vi "Main.vi"() -> ()   [LabVIEW 2017]
uses:
  types/Data Share Type.ctl
  E:/UPWORK/labview-offline-maps/labview/dll/OfflineMaps.Core.dll
  dll/OfflineMaps.Core.dll
  E:/UPWORK/labview-offline-maps/labview/dll/OfflineMaps.Controls.dll
  dll/OfflineMaps.Controls.dll
panel:
  in  "Load Button":bool
  in  "Temperature Alarm":dbl=25.0 caption="Alarm when temperature over, C"
  in  "Track file":path caption="Track file path:"
  in  "Map folder":path caption="Map folder path:"
  in  "Exit Button":bool
  in  "OfflineMapControl":refnum<k24>(container)
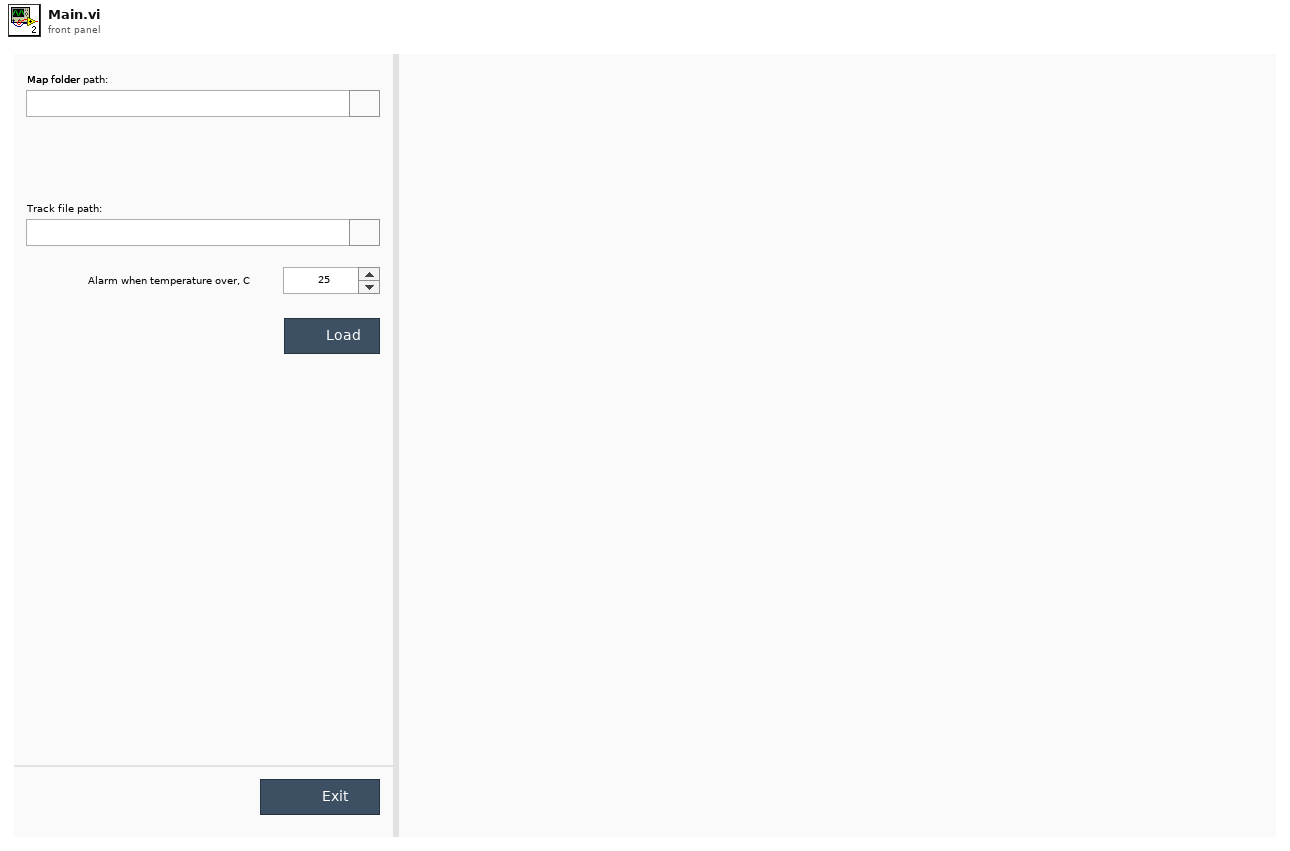
[diagram p1: front panel]
types:
  T1 = typedef "Data Share Type.ctl" = cluster{"Map folder":path, "Track file":path, "Latitude, deg:":dbl, "Longitude, deg:":dbl}
  T2 = cluster{"Warning":bool, "Caption":string, "Latitude_deg":dbl, "Longitude_deg":dbl, "Altitude_m":dbl, "Speed_m_s":dbl, "Temperature_C":dbl}[]
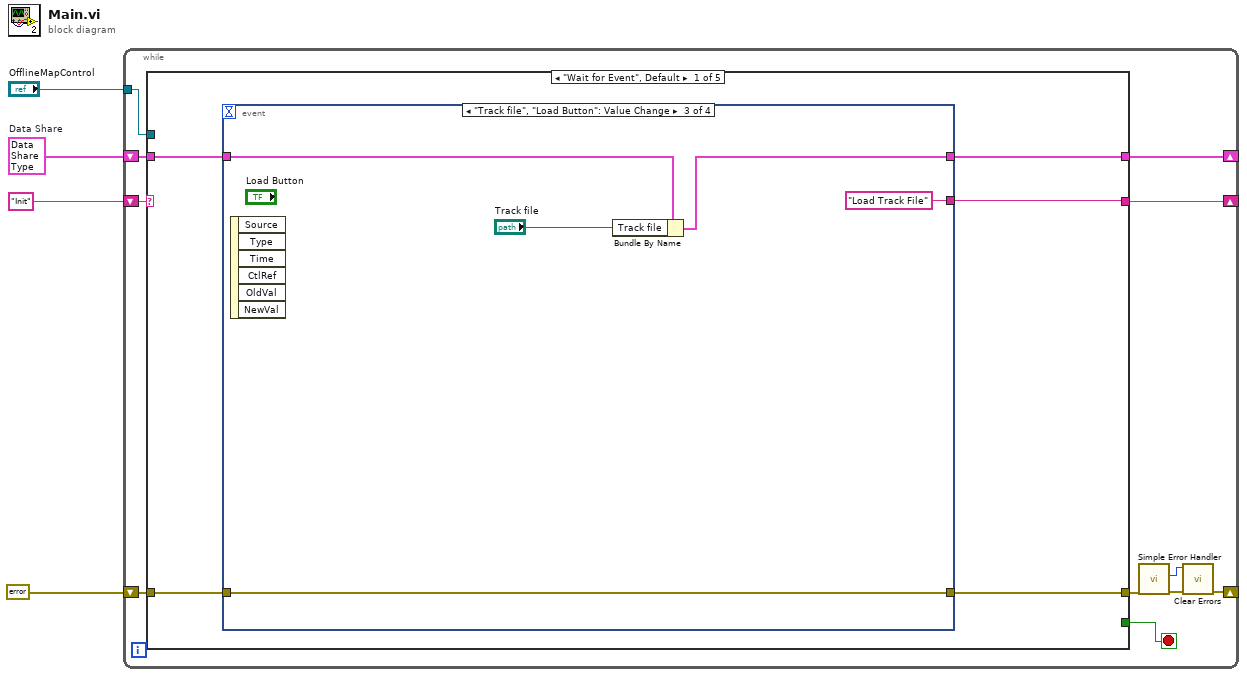
[diagram p0: block diagram]
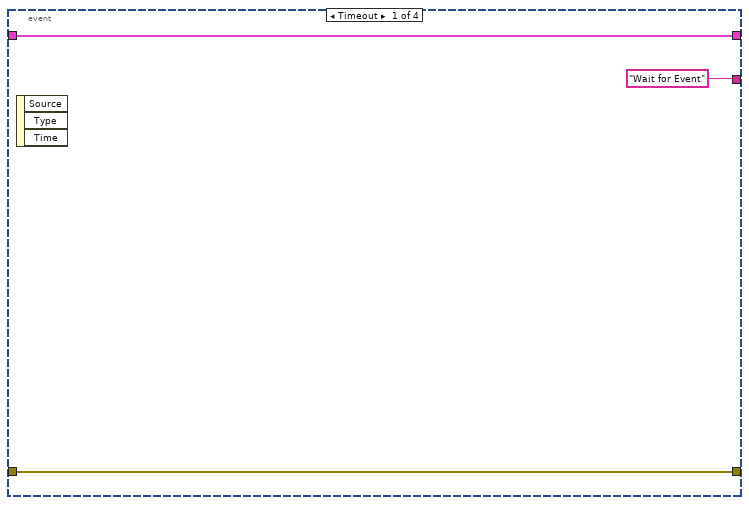
[diagram p2: hidden frame]
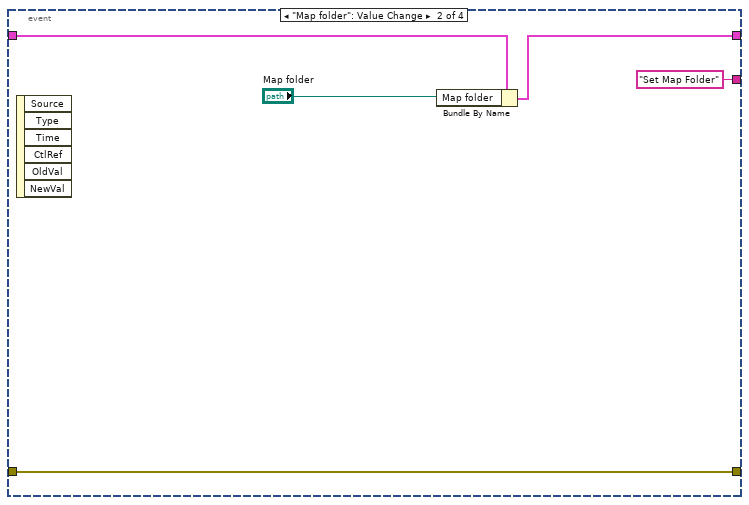
[diagram p3: hidden frame]
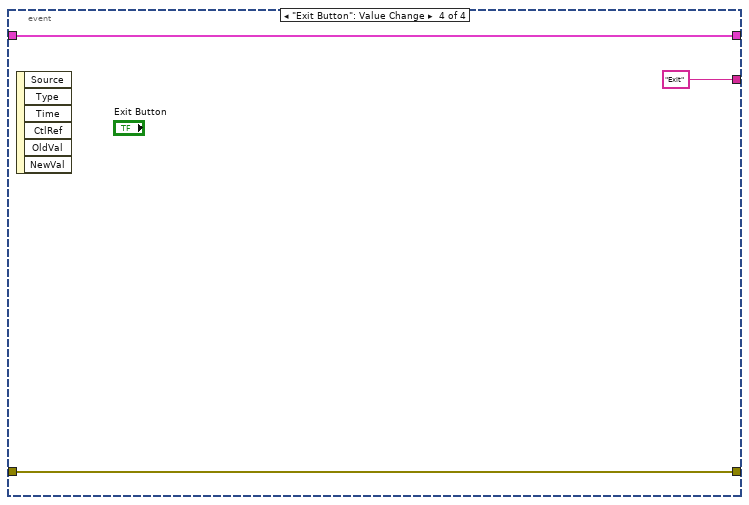
[diagram p4: hidden frame]
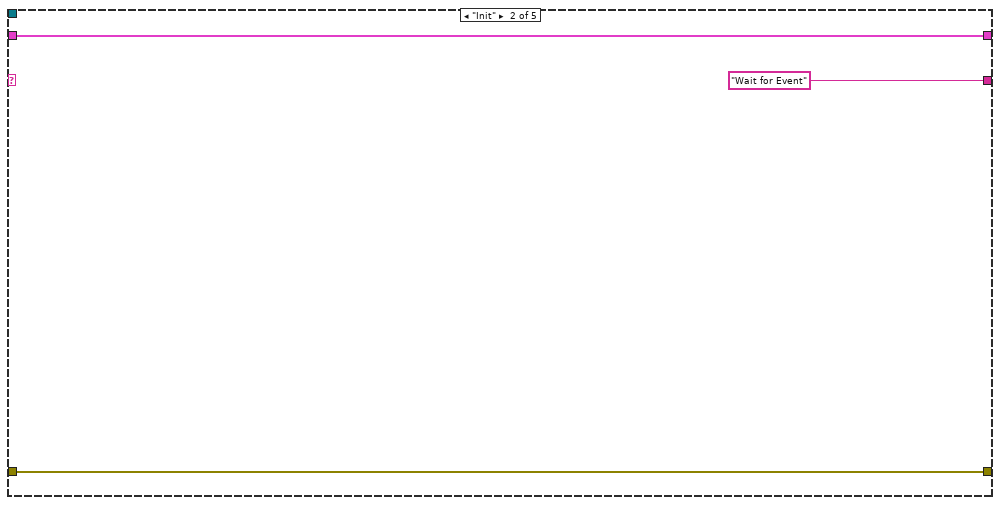
[diagram p5: hidden frame]
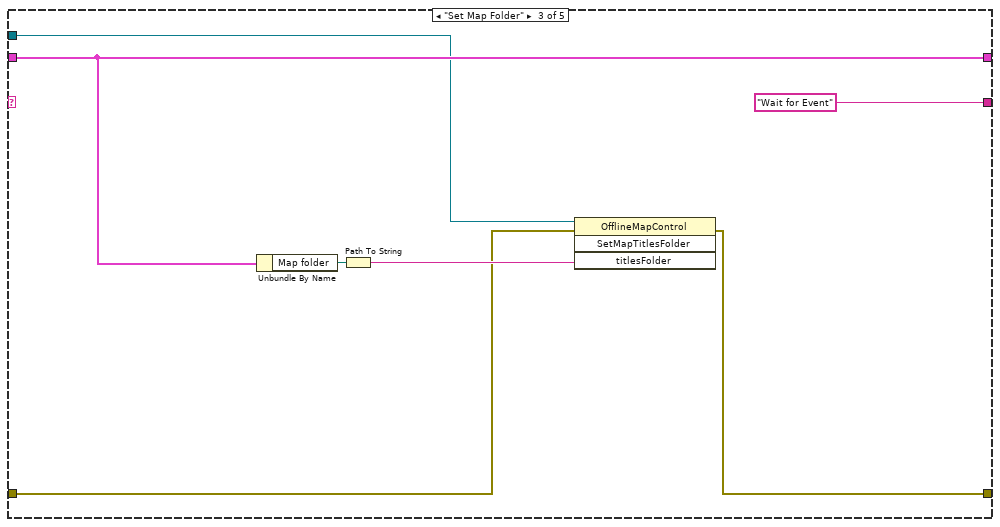
[diagram p6: hidden frame]
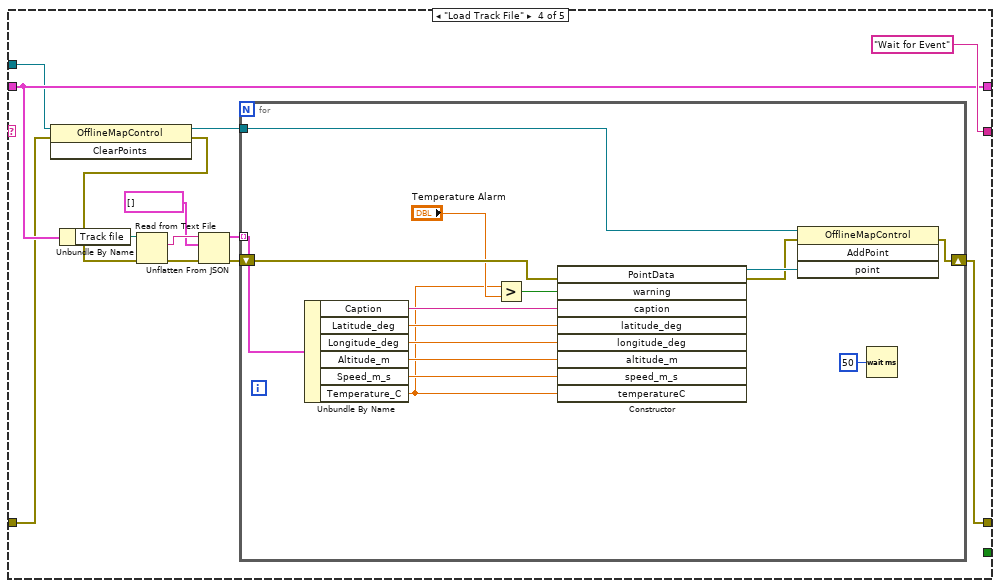
[diagram p7: hidden frame]
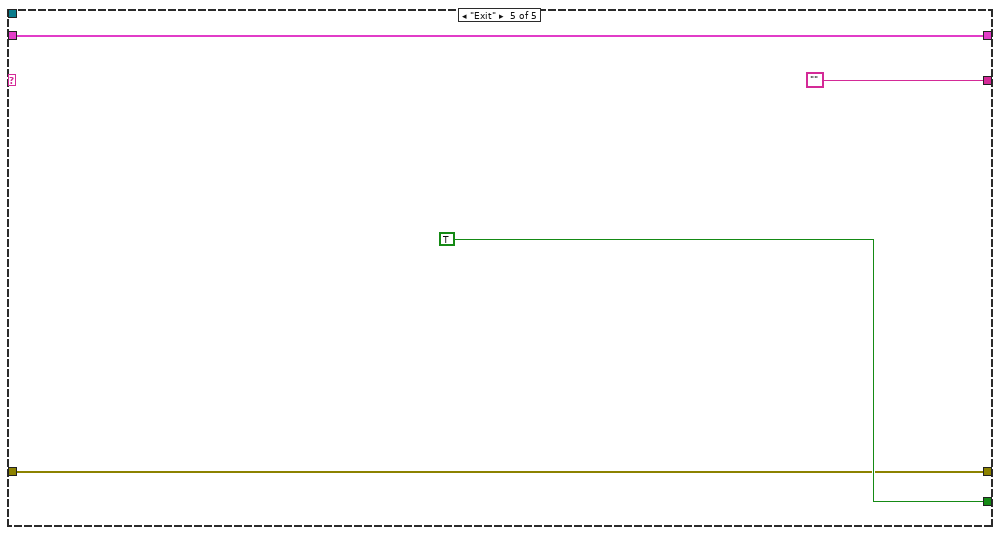
[diagram p8: hidden frame]
diagram:
  w3 = T1 {"Map folder"=path "", "Track file"=path "", "Latitude, deg:"=53.907767, "Longitude, deg:"=27.559764}  # Data Share
  n1 = while {
    shift-right: [w14] -> _
    shift-left: "Init" -> [w15]
    shift-right: [w11] -> _
    shift-left: w3 -> [w12]
    shift-right: [w6] -> _
    shift-left: errorcluster {"status"=FALSE, "code"=0, "source"=""} ("error in (no error)") -> [w10]
    tunnel: "OfflineMapControl" -> [w5]
    stop <- w13 stop-if-true
    n2 = case shown="\"Wait for Event\", Default" w15 {
      tunnel: [w20 "Wait for Event" "Wait for Event" "Wait for Event" ""] -> w14
      tunnel: [_ _ _ _ TRUE] -> w13
      tunnel: w12 -> [w19 w38 w45 w56 w76]
      tunnel: [w18 w38 w45 w56 w76] -> w11
      tunnel: w10 -> [w17 w37 w41 w48 w75]
      tunnel: [w16 w37 w40 w51 w75] -> w9
      tunnel: w5 -> [_ _ w43 w50 _]
      frame "Wait for Event", Default {
        n3 = event shown="[2] \"Track file\", \"Load Button\": Value Change" {
          selector: _ -> [_ _ _ _]
          dyn-events: _ -> [_ _ _ _]
          timeout: _ -> [_ _ _ _]
          tunnel: ["Wait for Event" "Set Map Folder" "Load Track File" "Exit"] -> w20
          tunnel: [w22 w27 w31 w35] -> w18
          tunnel: w19 -> [w22 w28 w32 w35]
          tunnel: w17 -> [w21 w24 w29 w34]
          tunnel: [w21 w24 w29 w34] -> w16
          event Timeout {
            n4 = event-data() -> ()  [unwired: 1 in, 3 out]
          }
          event "Map folder": Value Change {
            n5 = event-data() -> ()  [unwired: 1 in, 6 out]
            n6 = Bundle By Name(cluster=w28, "Map folder"="Map folder") -> (w27:T1)
          }
          event "Track file", "Load Button": Value Change {
            n7 = event-data() -> ()  [unwired: 1 in, 6 out]
            n8 = Bundle By Name(cluster=w32, "Track file"="Track file") -> (w31:T1)
          }
          event "Exit Button": Value Change {
            n9 = event-data() -> ()  [unwired: 1 in, 6 out]
          }
        }
      }
      frame "Init" {
      }
      frame "Set Map Folder" {
        n10 = Unbundle By Name(w45) -> ("Map folder"=w44:path)
        n11 = Path To String(path=w44) -> (string=w42:string)
        n12 = invoke class="OfflineMapControl" method="SetMapTitlesFolder"(reference=w43, error in=w41, "titlesFolder"=w42) -> (error out=w40:errorcluster)  [unwired: 1 in, 3 out]
      }
      frame "Load Track File" {
        n13 = invoke class="OfflineMapControl" method="ClearPoints"(reference=w50, error in=w48) -> (reference out=w49:refnum<k24>, error out=w47:errorcluster)  [unwired: 1 in, 1 out]
        n14 = Unbundle By Name(w56) -> ("Track file"=w55:path)
        n15 = Read from Text File(file (use dialog)=w55, error in=w47) -> (text=w58:string, error out=w54:errorcluster)  [unwired: 2 in, 2 out]
        n16 = Unflatten From JSON(JSON string=w58, type and defaults=T2 [], error in (no error)=w54) -> (value=w53:T2, error out=w52:errorcluster)  [unwired: 4 in]
        n17 = for {
          tunnel: w53 -> [w71] mode=indexing
          shift-right: [w72] -> w51
          shift-left: w52 -> [w70]
          tunnel: w49 -> [w67]
          n18 = Unbundle By Name(w71) -> ("Caption"=w65:string, "Latitude_deg"=w64:dbl, "Longitude_deg"=w63:dbl, "Altitude_m"=w62:dbl, "Speed_m_s"=w61:dbl, "Temperature_C"=w60:dbl)
          n19 = Greater?(x=w60, y="Temperature Alarm") -> (0:w66:bool)
          n20 = constructor class="OfflineMaps.Core.PointData"(error in=w70, "warning"=w66, "caption"=w65, "latitude_deg"=w64, "longitude_deg"=w63, "altitude_m"=w62, "speed_m_s"=w61, "temperatureC"=w60) -> (reference out=w74:refnum<k24>, error out=w73:errorcluster)  [unwired: 2 in, 8 out]
          n21 = invoke class="OfflineMapControl" method="AddPoint"(reference=w67, error in=w73, "point"=w74) -> (error out=w72:errorcluster)  [unwired: 1 in, 3 out]
          n22 = Wait (ms)(milliseconds to wait=u32 50) -> ()  [unwired: 1 out]
        }
      }
      frame "Exit" {
      }
    }
    n23 = call <vilib>:"Simple Error Handler.vi"("error in (no error)"=w9) -> ("code out"=w7:i32, "error out"=w8:errorcluster)  [unwired: 4 in, 3 out]
    n24 = call <vilib>:"Clear Errors.vi"("error in (no error)"=w8, "specific error code to clear (0: all)"=w7) -> ("error out"=w6:errorcluster)  [unwired: 4 in, 1 out]
  }
